vi "ParseMatlabParamName.vi"(10 "curNameIndex":i32, 11 "NamePath":string[](array[string])) -> (0 "At last name":bool, 1 "IsValidNameIndex":bool, 2 "Array Index (or -1)":i32, 3 "Name":string)   [LabVIEW 2017]
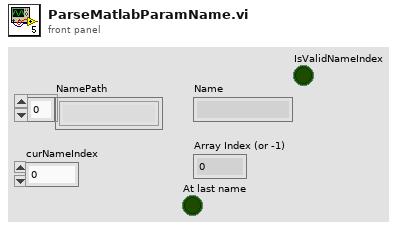
[diagram p1: front panel]
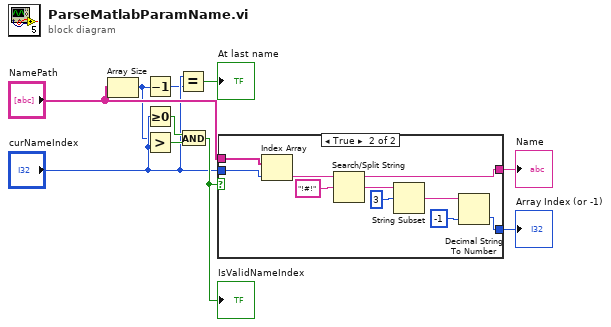
[diagram p0: block diagram]
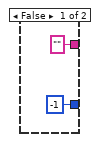
[diagram p2: hidden frame]
diagram:
  n1 = Array Size(array="NamePath") -> (size(s)=w1:i32)
  n2 = Decrement(x=w1) -> (x-1=w2:i32)
  n3 = Greater Or Equal To 0?(x="curNameIndex") -> (x >= 0?=w6:bool)
  n4 = Greater?(x=w1, y="curNameIndex") -> (0:w7:bool)
  n5 = Equal?(x="curNameIndex", y=w2) -> (x = y?=→"At last name":bool)
  n6 = And(x=w6, y=w7) -> (x .and. y?=w5:bool)
  "IsValidNameIndex" <- w5
  n7 = case shown="True" w5 {
    tunnel: "NamePath" -> [_ w19]
    tunnel: "curNameIndex" -> [_ w18]
    tunnel: ["" ("Name") w17] -> w10
    tunnel: [-1 w13] -> w9
    frame False {
    }
    frame True {
      n8 = Index Array(array=w19, index=w18) -> (element=w15:string)
      n9 = Search/Split String(string=w15, search string/char (-)="!#!") -> (substring before match=w17:string, match + rest of string=w21:string)  [unwired: 1 in, 1 out]
      n10 = String Subset(string=w21, offset (0)=3 ("length (rest)")) -> (substring=w22:string)  [unwired: 1 in]
      n11 = Decimal String To Number(string=w22, default (0L)=-1 ("default (0 I32)")) -> (number=w13:i32)  [unwired: 1 in, 1 out]
    }
  }
  "Name" <- w10
  "Array Index (or -1)" <- w9
